vi "Tool Data.GetPrivateEvents.vi"(8 "error in (no error)":errorcluster, 11 "Tool Data":refnum<class "Tool Data.lvclass">) -> (0 "error out":errorcluster, 2 "Private Events":T1, 3 "Tool Data out":refnum<class "Tool Data.lvclass">)   [LabVIEW 2019, in "Tool Data.lvclass"]
doc: "---------------------------------------------------------------\nJKI State Machine Objects™\nhttp://jki.net/state-machine-objects/\nCopyright (C) 2005-2015, JKI <info@jki.net>\nALL RIGHTS RESERVEDJKI State Machine Objects (SMO) 1.0.0.4\nJKI - JKI\nCopyright (c) 2015, JKI"
uses:
  Tool Data.lvclass
  Typedefs/PrivateEvents--Cluster.ctl
  Typedefs/PrivateEvents--Tool Data.Update Objects.ctl
  Settings/Setting Database/Typedefs/PublicEvents--Setting Database.PathsUpdated.ctl
  Settings/Path Settings/Path Settings.lvclass
  Settings/Setting Database/Typedefs/PublicEvents--Setting Database.RectanglesUpdated.ctl
  Settings/Rectangle Settings/Rectangle Settings.lvclass
  Settings/Setting Database/Typedefs/PublicEvents--Setting Database.FunnelsUpdated.ctl
  Settings/Funnel Settings/Funnel Settings.lvclass
  Settings/Setting Database/Typedefs/PublicEvents--Setting Database.DotsUpdated.ctl
  Settings/Dot Settings/Dot Settings.lvclass
  Parse/ParsePaths/Path.lvclass
  Parse/Rectangle/Rectangle.lvclass
  Parse/Image/SVGImage.lvclass
  Parse/Dot/Dot.lvclass
  Tool Data.lvclass/Tool Data.ctl
  Settings/Setting Database/Setting Database.lvclass
panel:
  # "For instructions on how to use the JKI State Machine Objects, examples and video tutorials, visit:\nhttp://jki.net/state-machine-objects/\n\nJKI State Machine Objects™\nhttp://jki.net/state-machine-objects/\nCopyright (C) 2005-2015, JKI <info@jki.net>\nALL RIGHTS RESERVED"
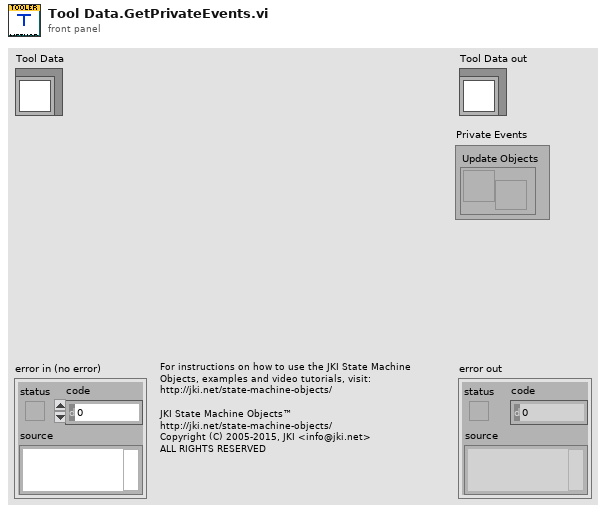
[diagram p1: front panel]
types:
  T1 = typedef "Tool Data.lvclass/PrivateEvents--Cluster.ctl" = cluster{"Update Objects":refnum<user-event>}
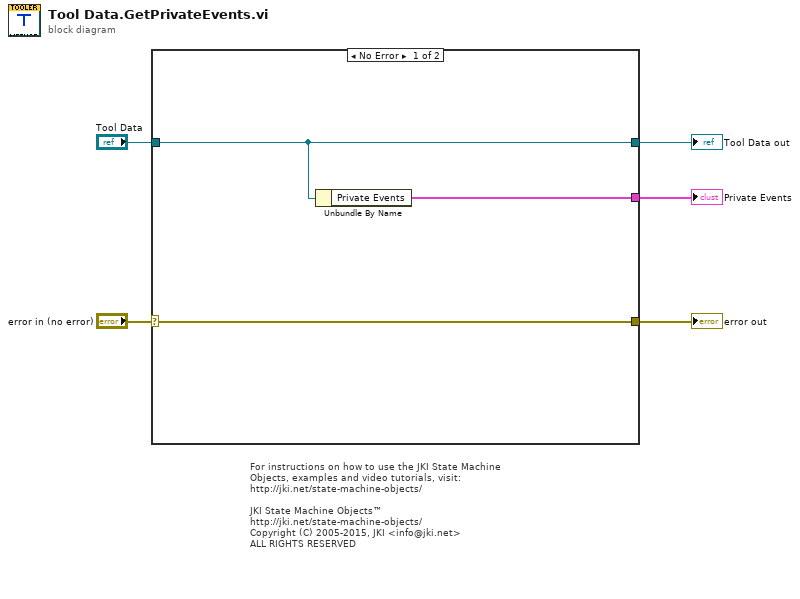
[diagram p0: block diagram]
diagram:
  # "For instructions on how to use the JKI State Machine Objects, examples and video tutorials, visit:\nhttp://jki.net/state-machine-objects/\n\nJKI State Machine Objects™\nhttp://jki.net/state-machine-objects/\nCopyright (C) 2005-2015, JKI <info@jki.net>\nALL RIGHTS RESERVED"
  n1 = case shown="No Error" "error in (no error)" {
    selector: "error in (no error)" -> [w7 w9]
    tunnel: "Tool Data" -> [w6 w10]
    tunnel: [w7 w9] -> w4
    tunnel: [w6 w10] -> w3
    tunnel: [w8 _] -> w1
    frame No Error {
      n2 = Unbundle By Name(w6) -> ("Private Events"=w8:T1)
    }
    frame Error {
    }
  }
  "error out" <- w4
  "Tool Data out" <- w3
  "Private Events" <- w1
